vi "PH_PowerUnit_BaseClass.String to SM State.vi"(1 "SM State String":string) -> (0 "SM State":T1)   [LabVIEW 2014, in "PH_PowerUnit_BaseClass.lvlib"]
uses:
  PH_PowerUnit_BaseClass.lvlib
  PH_PowerUnit_BaseClass.SM States.ctl
panel:
  in  "SM State":T1
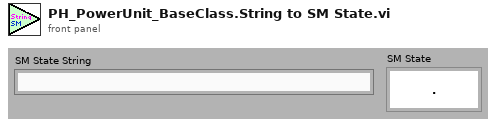
[diagram p1: front panel]
types:
  T1 = typedef "PH_PowerUnit_BaseClass.lvlib/PH_PowerUnit_BaseClass.SM States.ctl" = enum16{".", "Stand by", "Switch PU on", "Configure", "Set Default Voltage", "Set STANDBY", "Set READY", "Wait for Shot Cmd", "Open Dump Rods", "Open Ross Relais", "Close Ross Relais", "Switch PSU on", "Switch PSU off", "Charge", "Switch GD Channel on", "Close Dump Rods", "Rods-TO", "RR-TO", "PSU-TO", "Trigger-TO"}
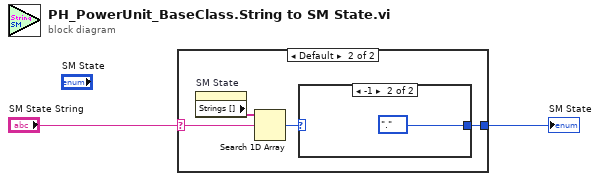
[diagram p0: block diagram]
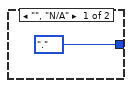
[diagram p2: hidden frame]
diagram:
  n1 = case shown="Default" "SM State String" {
    selector: "SM State String" -> [_ w4]
    tunnel: [PH_PowerUnit_BaseClass.SM_States."." ("SM State") w5] -> w1
    frame "", "N/A" {
    }
    frame Default {
      n2 = property on="SM State" class="Enum (strict)"() -> ("Strings []"=w7:string[])  [unwired: 2 in, 2 out]
      n3 = Search 1D Array(1D array=w7, element=w4) -> (index of element=w6:i32)  [unwired: 1 in]
      n4 = case shown="-1" w6 {
        selector: w6 -> [w8 _]
        tunnel: [w8 PH_PowerUnit_BaseClass.SM_States."." ("SM State")] -> w5
        frame Default {
        }
        frame -1 {
        }
      }
    }
  }
  "SM State" <- w1
